vi "Example Graph - AirPressure Callback.vi"(4 "AirPressure":refnum<user-event>, 5 "Event Data":cluster{"sender":refnum<k24>, "airPressure":i32}, 6 "Control Ref":refnum<k24>, 7 "Event Common Data":T1) -> ()   [LabVIEW 2010]
uses:
  C:/tf/play/labview/Tinkerforge.dll
  Tinkerforge.dll
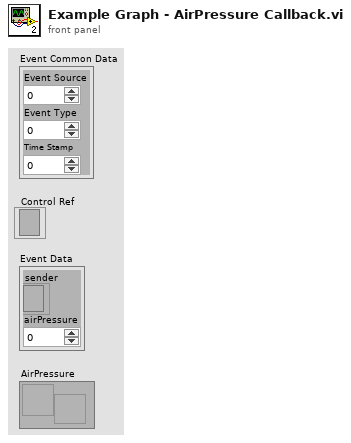
[diagram p1: front panel]
types:
  T1 = cluster{"Event Source":i32, "Event Type":u32, "Time Stamp":u32}
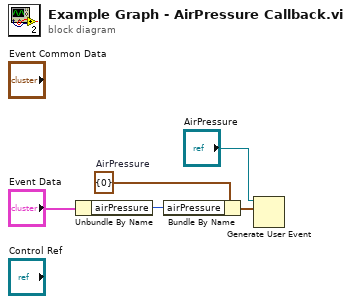
[diagram p0: block diagram]
diagram:
  w4 = cluster{"airPressure":i32} {"airPressure"=0}  # AirPressure
  n1 = Unbundle By Name("Event Data") -> ("airPressure"=w3:i32)
  n2 = Bundle By Name(cluster=w4, "airPressure"=w3) -> (w2:cluster{"airPressure":i32})
  n3 = Generate User Event(user event="AirPressure", event data cluster=w2) -> ()  [unwired: 1 in, 2 out]
